vi "GUI_CameraTriggers.vi"() -> ()   [LabVIEW 2020]
uses:
  Shared/GUI_Template/GUI_master/tcp_new_data_event.ctl
  Shared/GUI_Template/GUI_master/tcp new data cluster.ctl
  <userlib>/_OpenG.lib/array/array.llb/Search 1D Array (String)__ogtk.vi
  <userlib>/_OpenG.lib/array/array.llb/Index 1D Array Elements (String)__ogtk.vi
panel:
  in  "trigger::8":bool=TRUE caption="CAM-PL1-APLSideView"
  in  "exposure::8":dbl caption="CAM-PL1-APLSideView" min=3.8e-05 max=1.0
  in  "GUIdevice 8":string="CAM-PL1-APLSideView"
  in  "trigger::2":bool=TRUE caption="1BL-M1"
  in  "exposure::2":dbl caption="1BL-M1" min=3.8e-05 max=1.0
  in  "GUIdevice 2":string="CAM-1BL-M1"
  in  "exposure::33":dbl caption="CAM-PL1-TopView" min=1.0 max=50.0
  in  "exposure::31":dbl caption="SPEC-TEA-Qred"
  in  "exposure::30":dbl caption="SPEC-AA-Hamamastsu" min=1.0 max=300.0
  in  "exposure::21":dbl caption="CAM-TEA-MagSpecL" min=0.0001 max=1.0
  in  "exposure::20":dbl caption="CAM-TEA-MagSpecK" min=0.0001 max=1.0
  in  "exposure::19":dbl caption="CAM-TEA-MagSpecD" min=0.0001 max=1.0
  in  "exposure::18":dbl caption="CAM-TEA-MagSpecJ" min=0.0001 max=1.0
  in  "exposure::16":dbl caption="CAM-TEA-MagSpecI" min=0.0001 max=1.0
  in  "exposure::15":dbl caption="CAM-TEA-MagSpecH" min=0.0001 max=1.0
  in  "exposure::14":dbl caption="CAM-TEA-MagSpecG" min=0.0001 max=1.0
  in  "exposure::13":dbl caption="CAM-TEA-MagSpecC" min=0.0001 max=1.0
  in  "exposure::12":dbl caption="CAM-TEA-MagSpecB" min=0.0001 max=1.0
  in  "exposure::11":dbl caption="CAM-TEA-MagSpecA" min=0.0001 max=1.0
  in  "exposure::10":dbl caption="CAM-TEA-EBeam_Profile" min=3e-05 max=98990.0
  in  "exposure::9":dbl caption="CAM-PL1-SideSpec" min=2.5e-05 max=1.0
  in  "exposure::7":dbl caption="CAM-PL1-APLSideView" min=3.8e-05 max=1.0
  in  "exposure::6":dbl caption="CAM-HPD-HolyWedge" min=137.0 max=1000000.0
  in  "exposure::5":dbl caption="CAM-HPD-HeatCCD" min=3.8e-05 max=1.0
  in  "exposure::4":dbl caption="CAM-HPD-CCD" min=3.8e-05 max=1.0
  in  "exposure::3":dbl caption="CAM-1BL-M5" min=3.8e-05 max=1.0
  in  "exposure::1":dbl caption="1BL-M1" min=0.001 max=1.0
  in  "Trigger.mode::29":u16(ring)=2 caption="Trigger mode" items=["Auto", "Normal", "Single", "Single, auto trigger"]
  in  "Trigger.Slope::29":u16(ring) caption="Trigger Slope" items=["Rising", "Falling"]
  in  "Trigger.Source::29":u16(ring)=1 caption="Trigger Source" items=["Channel 1", "Channel 2", "Channel 3", "Channel 4", "External", "Power Line"]
  in  "Trigger.Level::29":dbl=0.04 caption="Trigger Level (V)" min=0.0001 max=30.0 format="%#_6p"
  in  "trigger::33":bool=TRUE caption="CAM-PL1-TopView"
  in  "GUIdevice 33":string="CAM-PL1-TopView"
  in  "Trigger.Mode::26":u16(ring) caption="DAQ-AA-3" items=["Immediate", "Analog Edge", "Analog Window", "Analog Hysteresis", "Video", "Digital Edge"]
  in  "Trigger.Mode::24":u16(ring) caption="DAQ-AA-2" items=["Immediate", "Analog Edge", "Analog Window", "Analog Hysteresis", "Video", "Digital Edge"]
  in  "Trigger.Mode::22":u16(ring) caption="DAQ-AA-1" items=["Immediate", "Analog Edge", "Analog Window", "Analog Hysteresis", "Video", "Digital Edge"]
  in  "trigger::31":bool=TRUE caption="SPEC-TEA-Qred"
  in  "trigger::30":bool=TRUE caption="SPEC-AA-Hamamastsu"
  in  "trigger::21":bool=TRUE caption="CAM-TEA-MagSpecL"
  in  "trigger::20":bool=TRUE caption="CAM-TEA-MagSpecK"
  in  "trigger::19":bool=TRUE caption="CAM-TEA-MagSpecJ"
  in  "trigger::18":bool=TRUE caption="CAM-TEA-MagSpecI"
  in  "trigger::16":bool=TRUE caption="CAM-TEA-MagSpecH"
  in  "trigger::15":bool=TRUE caption="CAM-TEA-MagSpecG"
  in  "trigger::14":bool=TRUE caption="CAM-TEA-MagSpecD"
  in  "trigger::13":bool=TRUE caption="CAM-TEA-MagSpecC"
  in  "trigger::12":bool=TRUE caption="CAM-TEA-MagSpecB"
  in  "trigger::11":bool=TRUE caption="CAM-TEA-MagSpecA"
  in  "trigger::10":bool=TRUE caption="CAM-TEA-EBeam_Profile"
  in  "trigger::9":bool=TRUE caption="CAM-PL1-SideSpec"
  in  "trigger::7":bool=TRUE caption="CAM-PL1-APLSideView"
  in  "trigger::6":bool=TRUE caption="CAM-HPD-HolyWedge"
  in  "trigger::5":bool=TRUE caption="CAM-HPD-HeatCCD"
  in  "trigger::4":bool=TRUE caption="CAM-HPD-CCD"
  in  "trigger::3":bool=TRUE caption="CAM-1BL-M5"
  in  "trigger::1":bool=TRUE caption="1BL-M1"
  in  "GUIdevice 31":string="SPEC-TEA-Qred"
  in  "GUIdevice 30":string="SPEC-AA-Hamamastsu"
  in  "Jet trigger":bool caption="Triggers"
  in  "GUIdevice 4":string="CAM-HPD-CCD"
  in  "GUIdevice 6":string="CAM-HPD-HolyWedge"
  in  "GUIdevice 29":string="SCOPE-AA-LeCroy8254M"
  in  "GUIdevice 26":string="DAQ-AA-3"
  in  "GUIdevice 24":string="DAQ-AA-2"
  in  "GUIdevice 22":string="DAQ-AA-1"
  in  "GUIdevice 21":string="CAM-TEA-MagSpecL"
  in  "GUIdevice 20":string="CAM-TEA-MagSpecK"
  in  "GUIdevice 19":string="CAM-TEA-MagSpecJ"
  in  "GUIdevice 18":string="CAM-TEA-MagSpecI"
  in  "GUIdevice 16":string="CAM-TEA-MagSpecH"
  in  "GUIdevice 15":string="CAM-TEA-MagSpecG"
  out "error IO 2":errorcluster
  out "tcp data event":T1
  in  "GUIdevice 14":string="CAM-TEA-MagSpecD"
  in  "GUIdevice 13":string="CAM-TEA-MagSpecC"
  in  "GUIdevice 7":string="CAM-PL1-APLSideView"
  in  "GUIdevice 10":string="CAM-TEA-EBeam_Profile"
  in  "GUIdevice 5":string="CAM-HPD-HeatCCD"
  in  "GUIdevice 1":string="CAM-1BL-M1"
  in  "GUIdevice 3":string="CAM-1BL-M5"
  in  "GUIdevice 11":string="CAM-TEA-MagSpecA"
  in  "GUIdevice 12":string="CAM-TEA-MagSpecB"
  in  "GUIdevice 9":string="CAM-PL1-SideSpec"
  in  "stop":bool
  # "CAM-1BL-CompG4\n\nCAM-1BL-M1back\n\n\n\nCAM-2BL-GHOST\n\n\n\nCAM-HPD-CCD2\nCAM-HPD-CCD3\n\nCAM-HPD-HeatM3\n\n\nCAM-LT-SPLIT\nCAM-LT-XPW\n\nCAM-PL1-LPMode\nCAM-PL1-PMReflect\n\nCAM-PL1-SideSpec\nCAM-PL1-SideView\nCAM-PL1-TopView\n\n\n\n\n\n\n\n\nCAM-TEA-MagSpecHR\n\n\n\n\n\n\n\nEM-HPD-1\nEM-LB-1\nEM-LB-1\nEM-LB-PL\nFROG-HPD-1\nFROG-LB-1\nHPD-Phasics151\nIP2-MCPcam\nIP2-modeim\nIP2-Reflected1\nIP2-Reflected1\nIP2-targetobs\nIP2-targetscatt\nIP2-transmit\nP2-AndorCam\nP2-DG535\nP2-HeatCamPost\nP2-HeatCamPostNear\nP2-HeatCamPreFar\nP2-HeatCamPreNear\nP2-HeatCamPreNear\nP2-HeatEnergy\nP2-HeatEnergy\nP2-phasics\nP2-phasicsHR\nP2-ProbeCamPost\nP2-ProbeCamPostNear\nP2-ProbeCamPreNear\nP2-SideView\nP2-SRS\nP2-SRS\nP2FastDiag645\nP2FastDiag645\n\nSCOPE-LT-LeCroy64Xi\nSCOPE-PL1-PXIfast\nSCOPE-PL1-PXIfast\nSCOPE-PL1-PXIfast\nSCOPE-PL1-PXIfast\nSPEC-AA-Hamamastsu\nSPEC-PL1-Thorlabs\nSPEC-TEA-Qred"
  # "BELLA Triggers"
  # "SCOPE-AA-LeCroy8254M"
  # "Trigger"
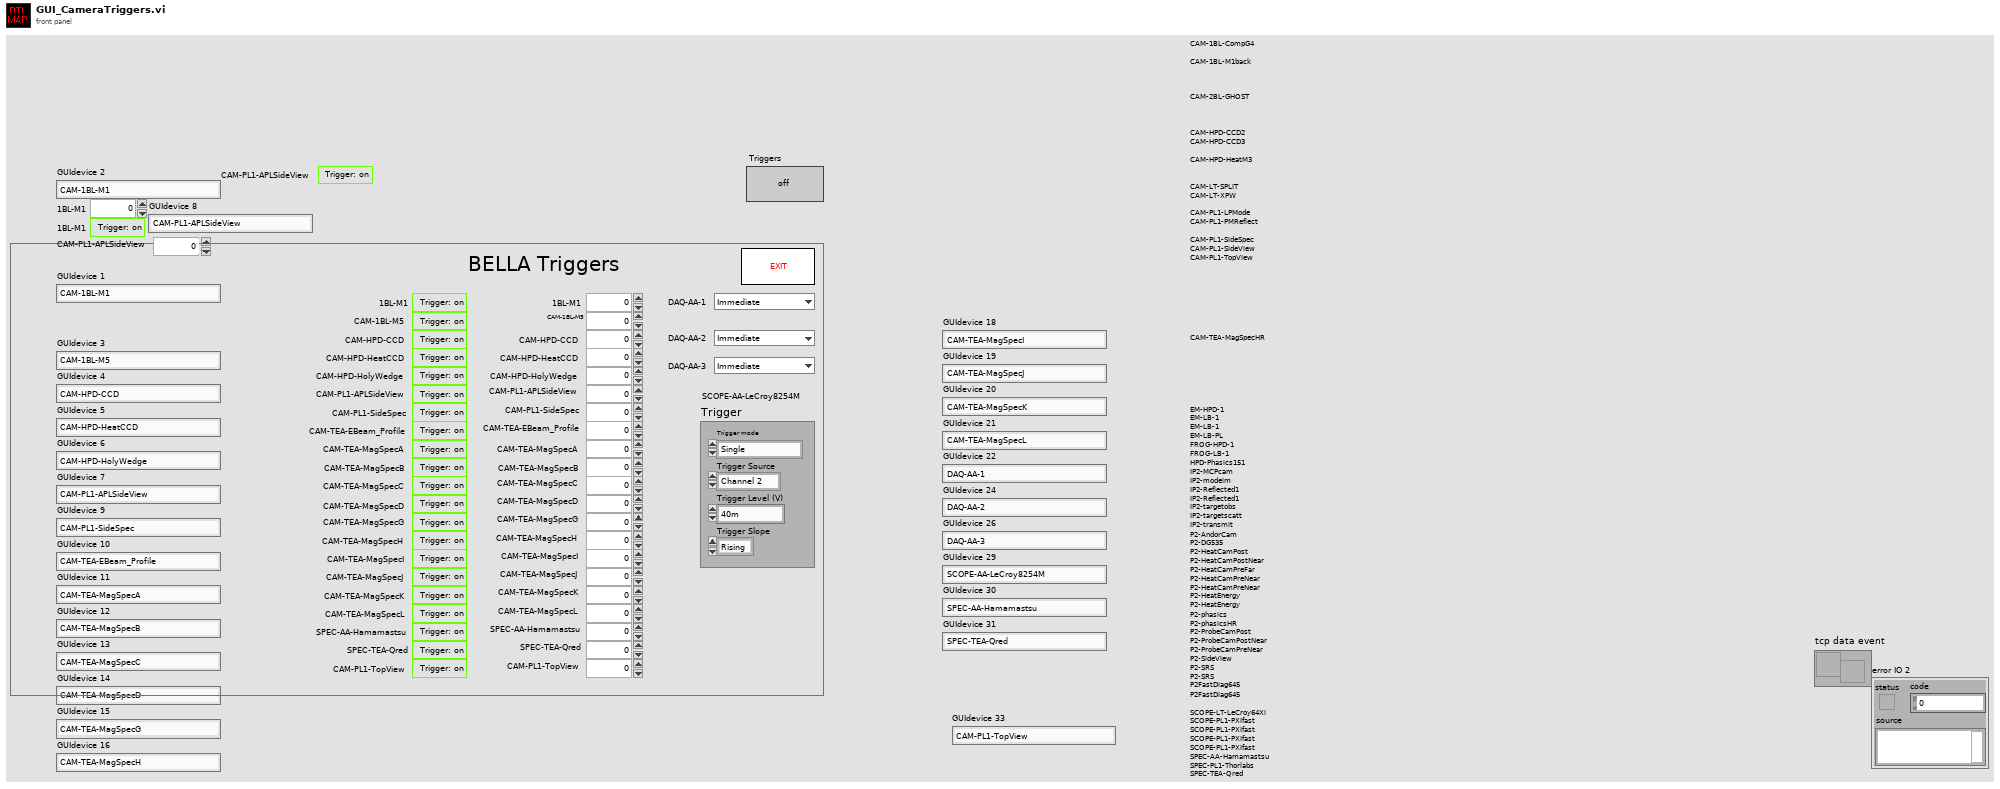
[diagram p1: front panel]
types:
  T1 = typedef "tcp_new_data_event.ctl" = refnum<user-event>
  T2 = typedef "tcp new data cluster.ctl" = cluster{"EventEnum":enum16{"new data", "connection status update"}, "Device name":string}
  T3 = enum32{"invalid app kind", "Development System", "Run Time System", "Student Edition", "Embedded LabVIEW", "Evaluation", "Custom"}
  T4 = enum32{"Invalid", "Standard", "Closed", "Hidden", "Minimized", "Maximized"}
  T5 = cluster{"Core":cluster{"Current VI Reference":refnum<vi>, "Close Panel on Exit?":bool}, "Heater timing offset":dbl, "Discharge timing offset":dbl, "Jet trigger":bool, "Tik1":u32, "Tik2":u32, "Fire Continues Allowed":bool}
  T6 = cluster{"Current VI Reference":refnum<vi>, "Close Panel on Exit?":bool}
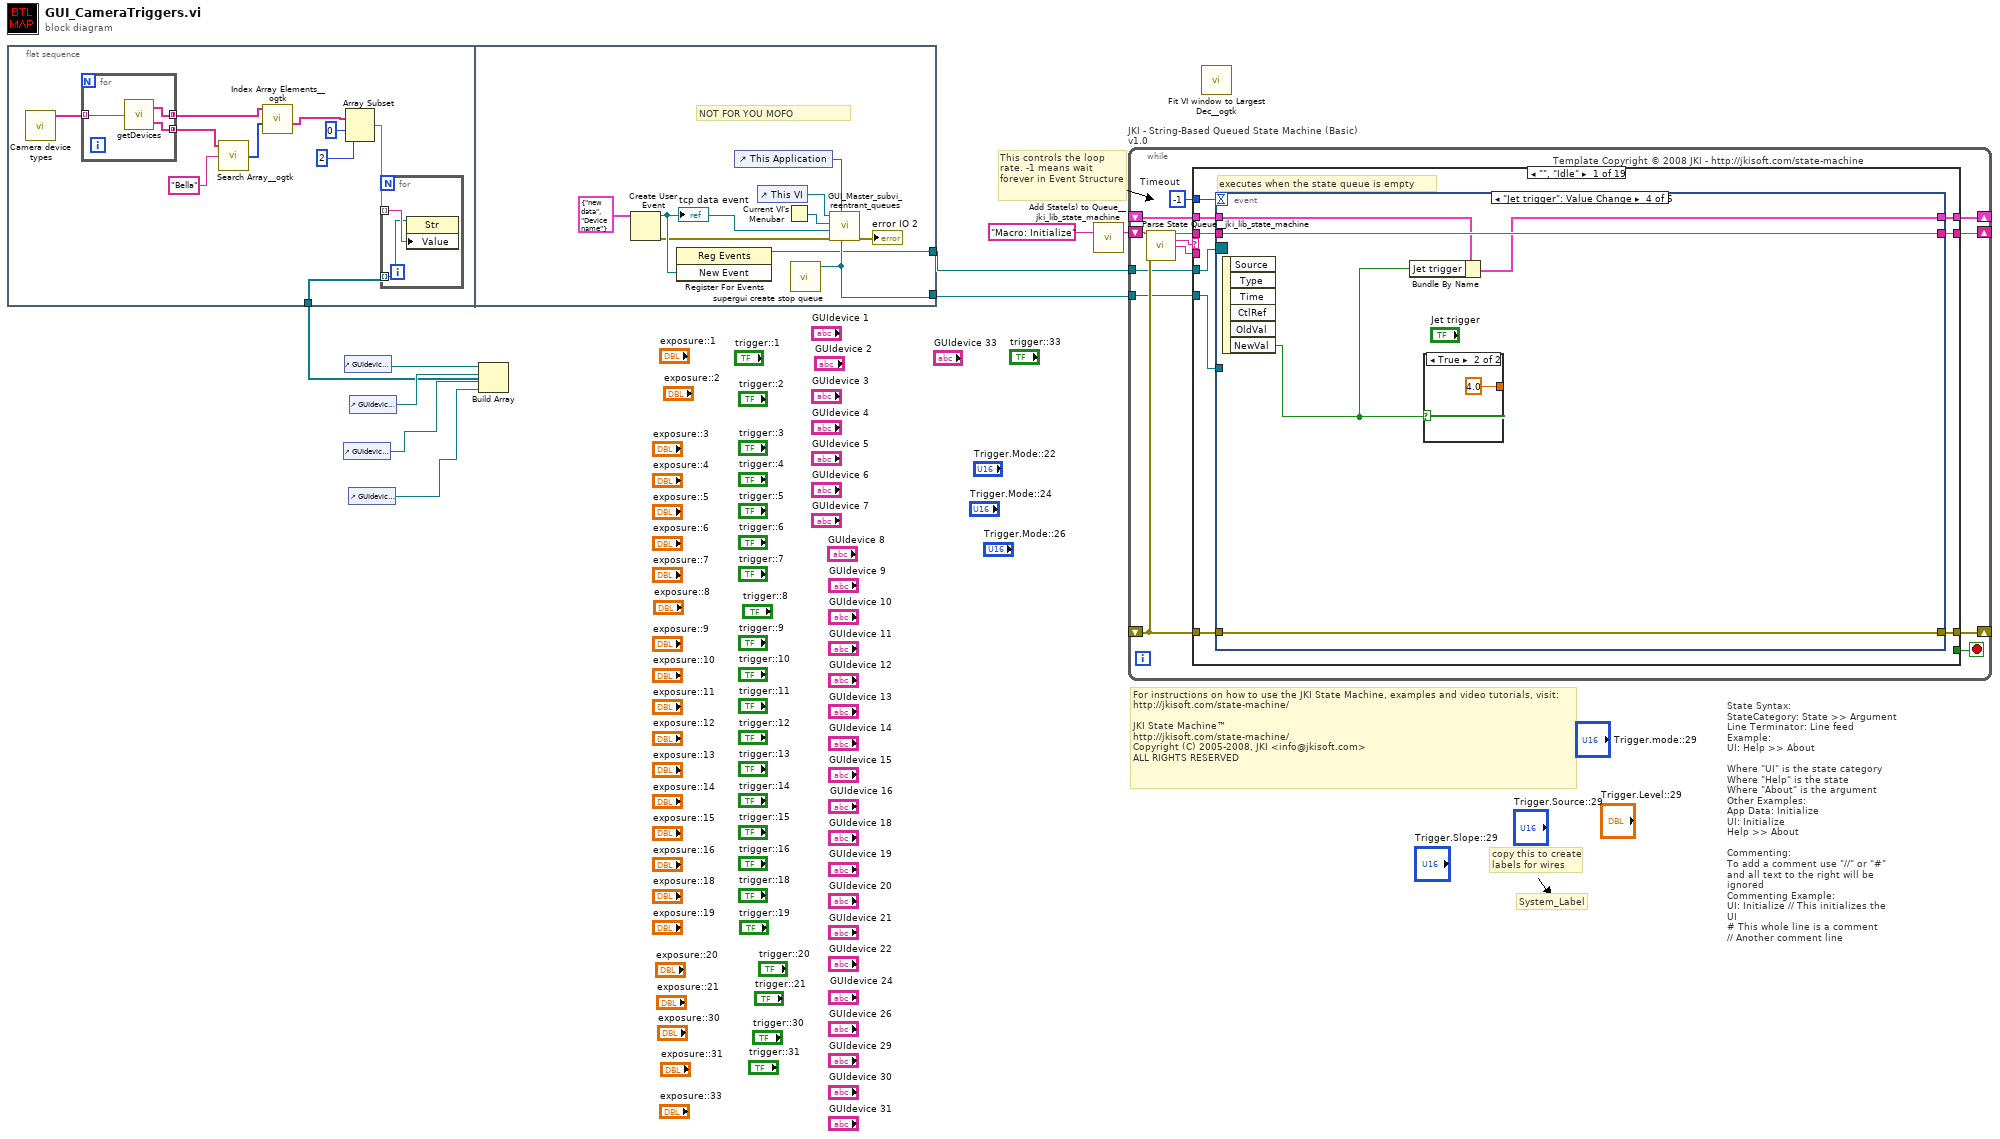
[diagram p0: block diagram]
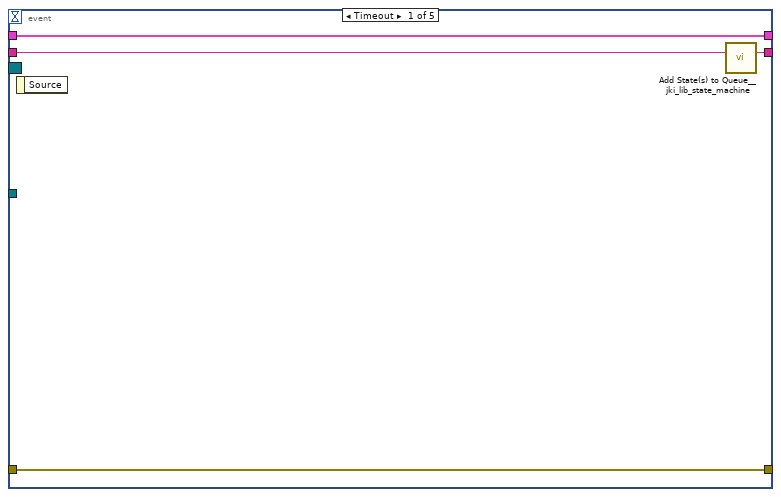
[diagram p2: hidden frame]
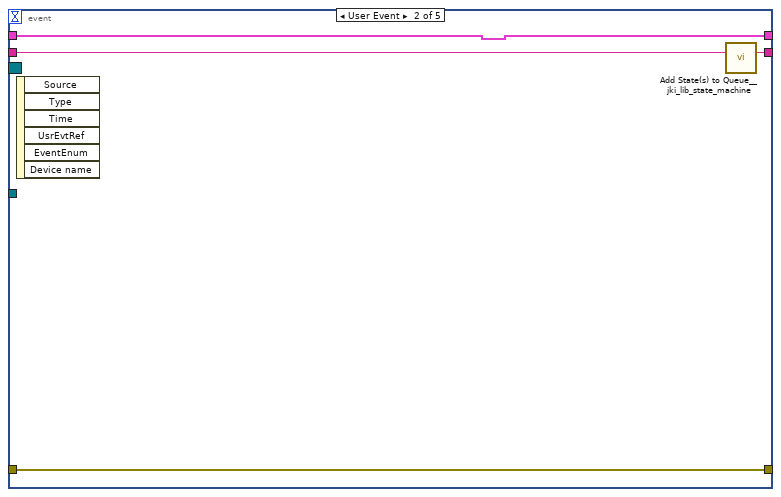
[diagram p3: hidden frame]
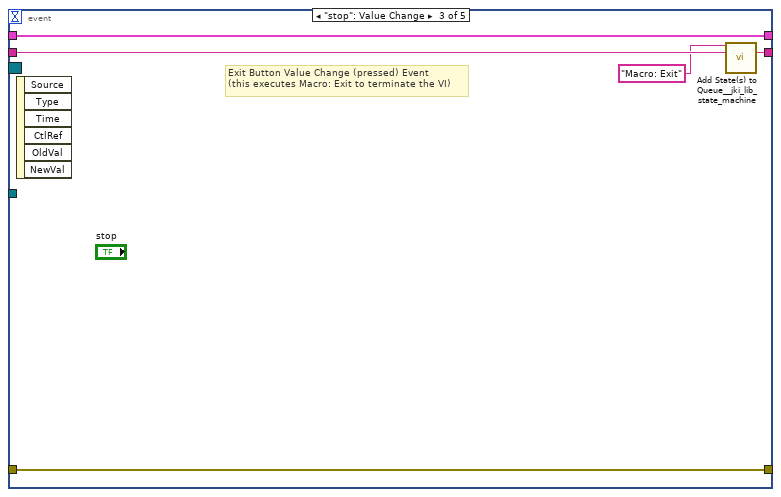
[diagram p4: hidden frame]
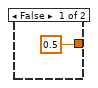
[diagram p5: hidden frame]
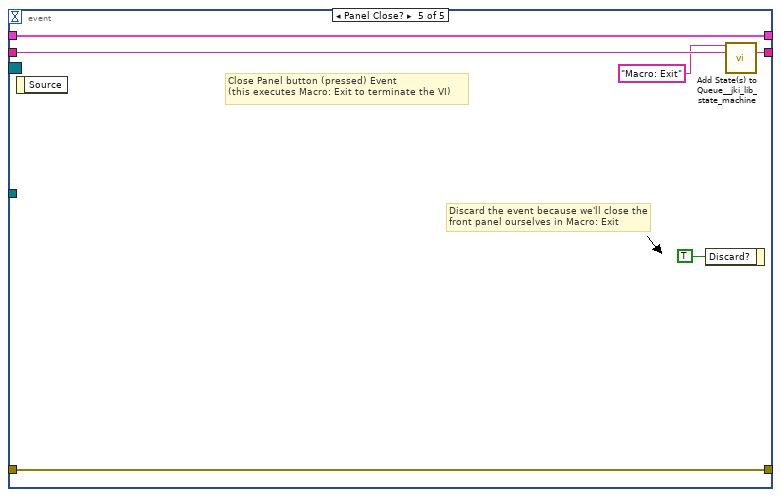
[diagram p6: hidden frame]
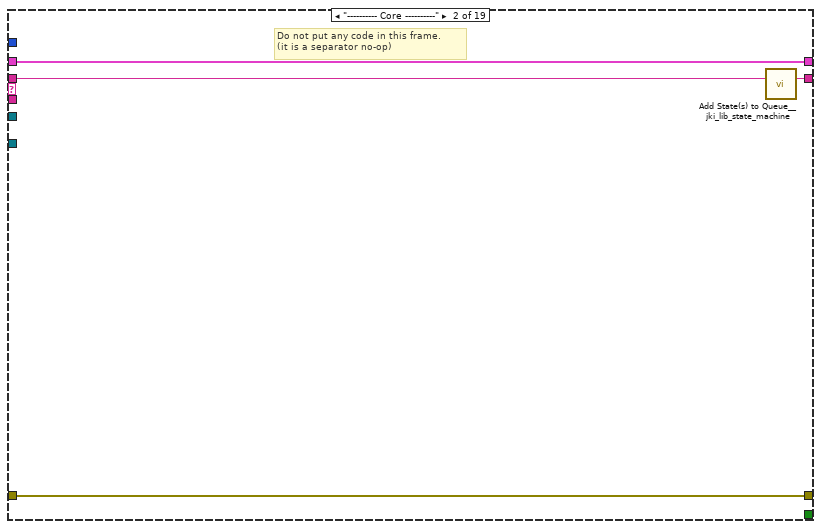
[diagram p7: hidden frame]
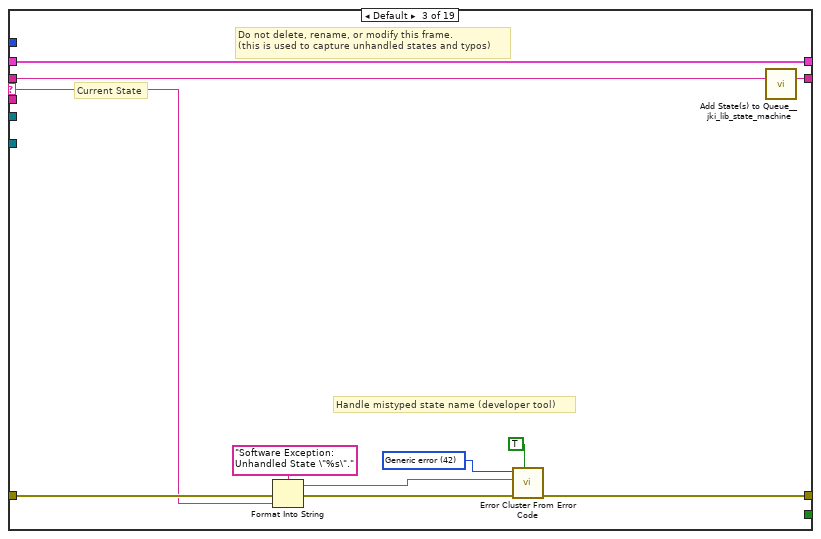
[diagram p8: hidden frame]
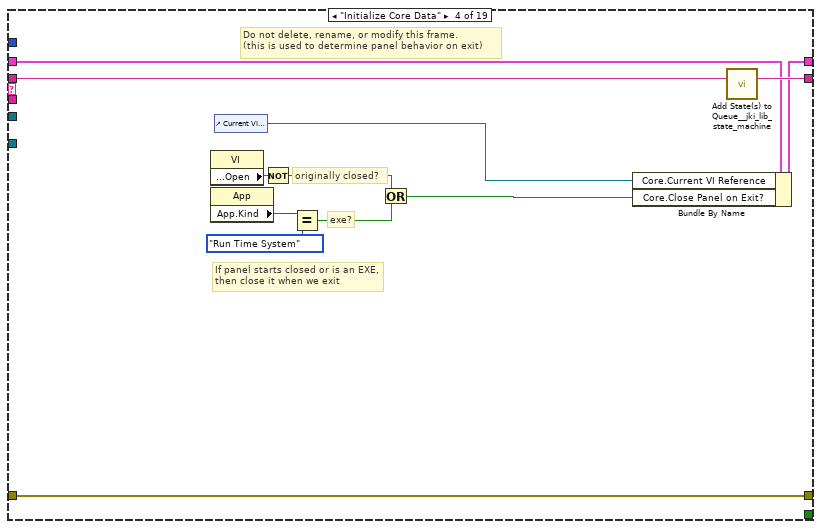
[diagram p9: hidden frame]
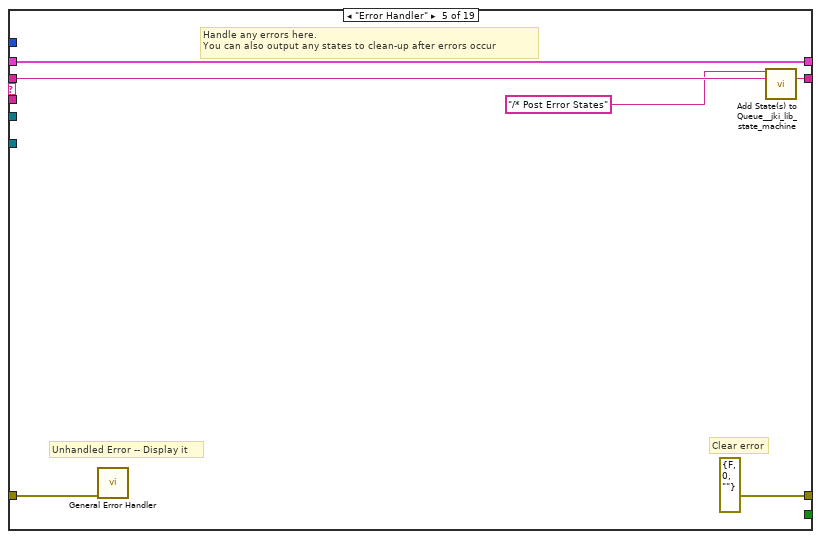
[diagram p10: hidden frame]
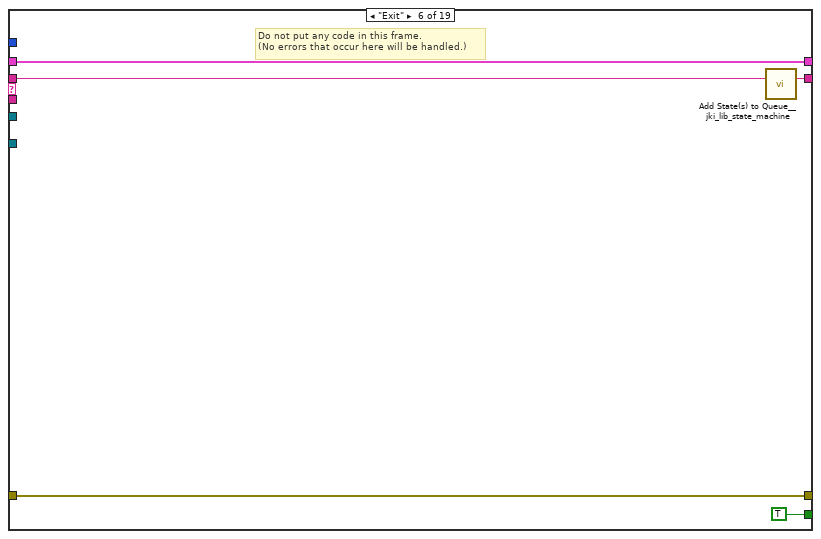
[diagram p11: hidden frame]
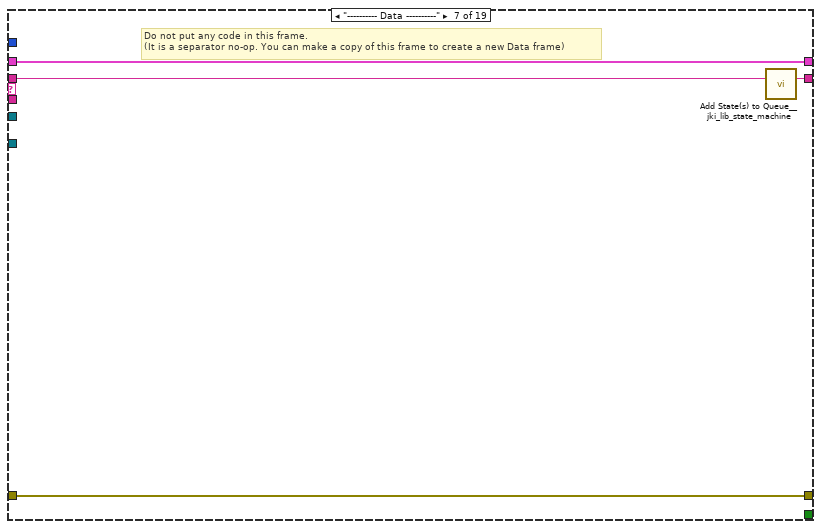
[diagram p12: hidden frame]
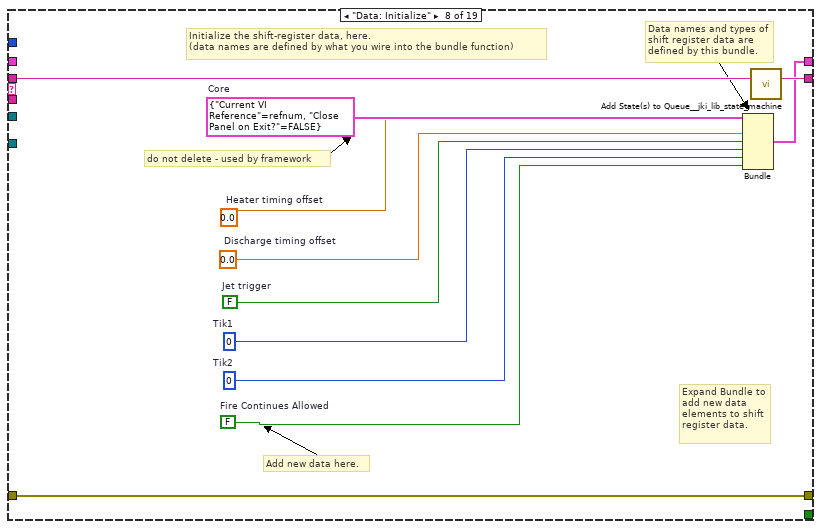
[diagram p13: hidden frame]
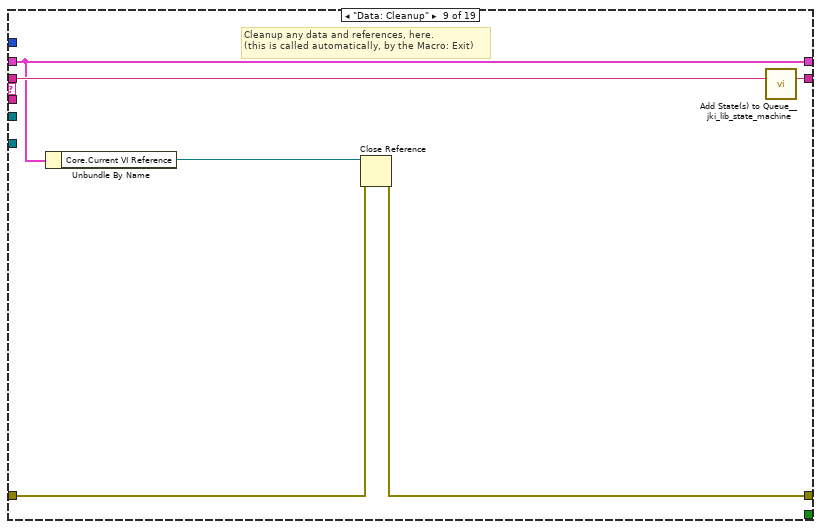
[diagram p14: hidden frame]
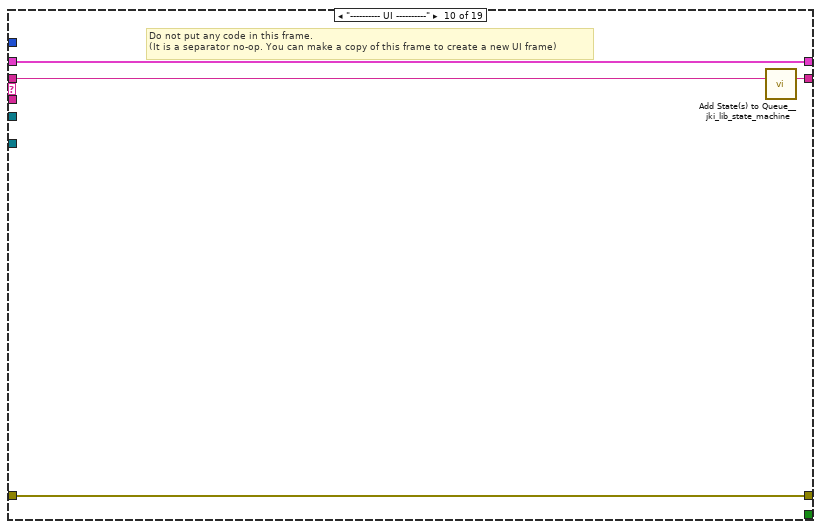
[diagram p15: hidden frame]
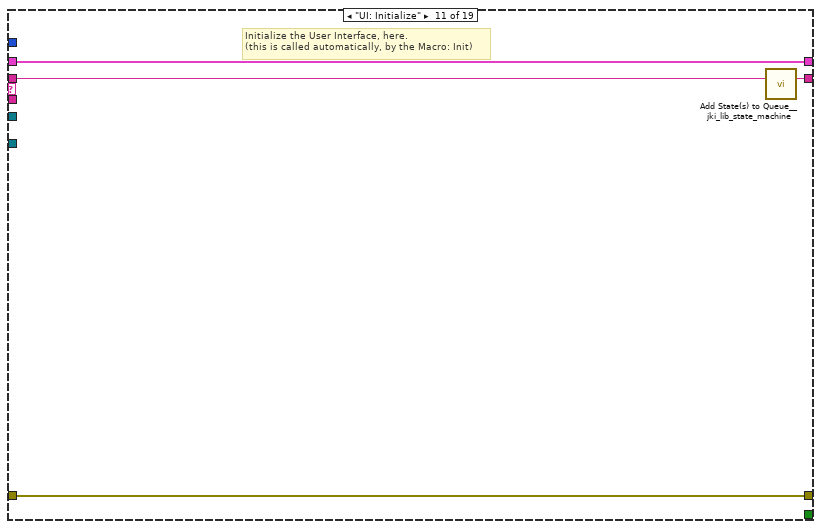
[diagram p16: hidden frame]
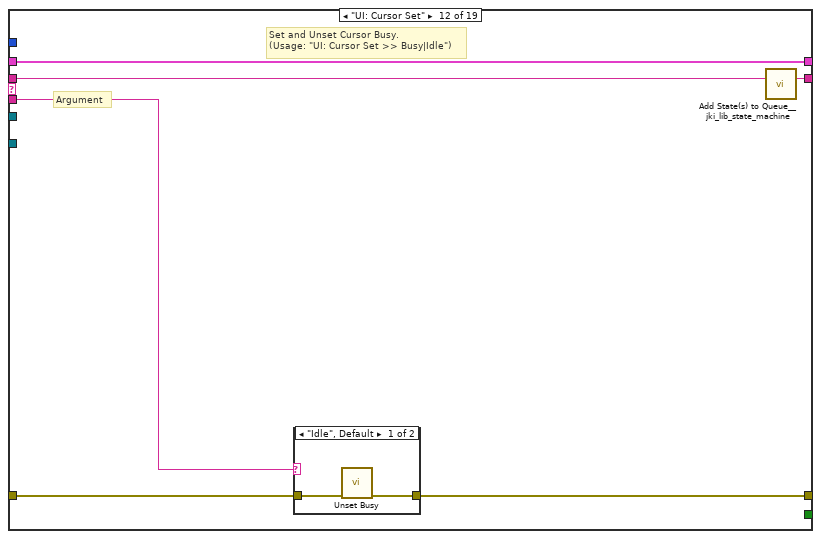
[diagram p17: hidden frame]
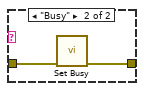
[diagram p18: hidden frame]
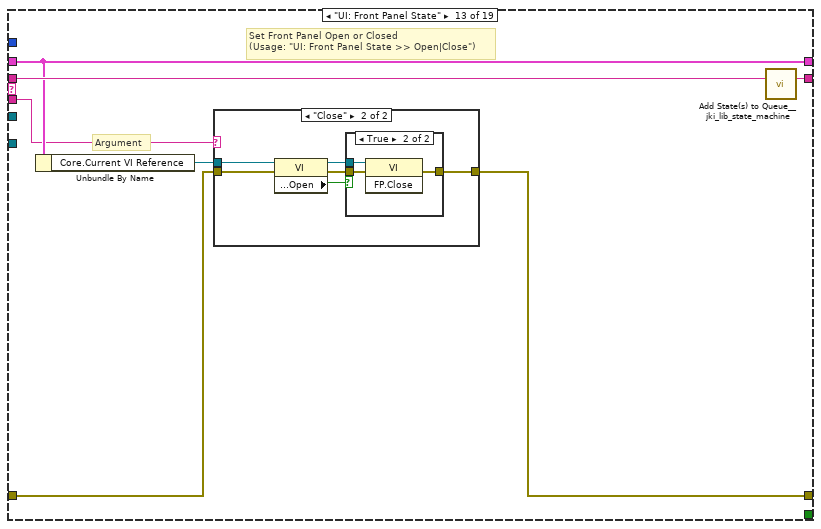
[diagram p19: hidden frame]
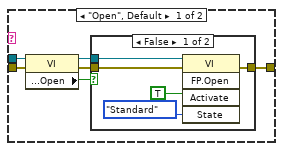
[diagram p20: hidden frame]
diagram:
  # "For instructions on how to use the JKI State Machine, examples and video tutorials, visit:\nhttp://jkisoft.com/state-machine/\n\nJKI State Machine™\nhttp://jkisoft.com/state-machine/\nCopyright (C) 2005-2008, JKI <info@jkisoft.com>\nALL RIGHTS RESERVED"
  # "State Syntax:\nStateCategory: State >> Argument\nLine Terminator: Line feed\nExample:\nUI: Help >> About\n\nWhere \"UI\" is the state category\nWhere \"Help\" is the state\nWhere \"About\" is the argument\nOther Examples:\nApp Data: Initialize\nUI: Initialize\nHelp >> About\n\nCommenting:\nTo add a comment use \"//\" or \"#\" and all text to the right will be ignored\nCommenting Example:\nUI: Initialize // This initializes the UI\n# This whole line is a comment\n// Another comment line"
  # "copy this to create labels for wires"
  # "This controls the loop rate. -1 means wait forever in Event Structure"
  # "System_Label"
  n1 = flat-sequence {
    tunnel: w1 -> [w15]
    tunnel: [w26] -> w7
    tunnel: [w25] -> w6
    frame #0 {
      n2 = call "Camera device types.vi"() -> ("Camera device types"=w19:string[])  [unwired: 11 in]
      n3 = for {
        tunnel: [w24] -> w12 mode=concatenating
        tunnel: w19 -> [w23] mode=indexing
        tunnel: [w22] -> w14 mode=concatenating
        n4 = call "getDevices.vi"("Device Class"=w23) -> ("All Devices"=w24:string[], "Expts"=w22:string[])
      }
      n5 = call-poly <userlib>:"Search Array__ogtk.vi"("Array"=w14, "Element Data"="Bella") -> ("Indices of Elements"=w11:i32[])  [unwired: 7 in]
      n6 = call-poly <userlib>:"Index Array Elements__ogtk.vi"("indices"=w11, "array"=w12) -> ("elements"=w10:string[])  [unwired: 9 in]
      n7 = Array Subset(array=w10, index=0, length=2) -> (w16:string[])
      n8 = for {
        tunnel: w16 -> [w21] mode=indexing
        tunnel: w15 -> [w20] mode=indexing
        n9 = property on="Property Node" class="Str"(reference=w20, "Value"=w21) -> ()  [unwired: 1 in, 2 out]
      }
    }
    frame #1 {
      # "NOT FOR YOU MOFO"
      n10 = Create User Event(user event datatype=T2 {"EventEnum"=enum."new data", "Device name"="Device name"} ("New Event")) -> (user event=w32:refnum<user-event>, error out=w31:errorcluster)  [unwired: 1 in]
      "tcp data event" <- w32
      n11 = register-events(w32) -> (reference out=w25:refnum<event-registration>)  [unwired: 2 in, 1 out]
      n12 = control-ref of="This Application"() -> (w33:refnum<vi>)
      n13 = control-ref of="This VI"() -> (w27:refnum<vi>)
      n14 = Current VI's Menubar() -> (w29:refnum<k9>)
      n15 = call "supergui create stop queue.vi"() -> ("STOP Queue out"=w26:refnum<queue>)  [unwired: 11 in]
      n16 = call "GUI_Master_subvi_reentrant_queues.vi"("STOP Queue in"=w26, "This Application"=w33, "error in (no error)"=w31, "tcp data event"=w32, "Caller menu reference"=w29, "Caller VI ref"=w27) -> ("error out"=→"error IO 2":errorcluster)  [unwired: 5 in]
    }
  }
  n17 = control-ref of="GUIdevice 3"() -> (w3:refnum<vi>)
  n18 = control-ref of="GUIdevice 1"() -> (w5:refnum<vi>)
  n19 = control-ref of="GUIdevice 4"() -> (w2:refnum<vi>)
  n20 = control-ref of="GUIdevice 2"() -> (w4:refnum<vi>)
  n21 = Build Array(w5, w4, w3, w2) -> (w1:refnum<vi>[])
  n22 = call <vilib>:"Add State(s) to Queue__jki_lib_state_machine.vi"("State(s) in (\"\")"="Macro: Initialize") -> ("States Out"=w8:string)  [unwired: 14 in]
  n23 = while "JKI - String-Based Queued State Machine (Basic) v1.0" {
    shift-right: [w39] -> _
    shift-left: _ -> [w38]
    shift-right: [w42] -> _
    shift-left: _ -> [w36]
    shift-right: [w41] -> _
    shift-left: w8 -> [w43]
    tunnel: w6 -> [w35]
    tunnel: w7 -> [w34]
    stop <- w40 stop-if-true
    w37 = -1  # Timeout
    # "Template Copyright © 2008 JKI - http://jkisoft.com/state-machine"
    n24 = call <vilib>:"Parse State Queue__jki_lib_state_machine.vi"("State Queue"=w43, "Error In (no error)"=w36) -> ("Remaining States"=w45:string, "Current State"=w46:string, "Arguments"=w44:string)  [unwired: 11 in]
    n25 = case shown="\"\", \"Idle\"" w46 {
      selector: w46 -> [_ _ w86 _ _ _ _ _ _ _ _ _ _ _ _ _ _ _ _]
      tunnel: w45 -> [w55 w85 w90 w108 w114 w119 w123 w134 w140 w144 w148 w154 w165 w191 w196 w209 w213 w225 w232]
      tunnel: w44 -> [_ _ _ _ _ _ _ _ _ _ _ w149 w159 _ _ _ _ _ _]
      tunnel: w38 -> [w53 w82 w88 w99 w111 w117 w120 _ w135 w141 w146 w152 w161 w188 w193 w206 w210 w222 w230]
      tunnel: [w52 w83 w92 w105 errorcluster {"status"=FALSE, "code"=0, "source"=""} ("error out") w116 w121 w131 w136 w142 w145 w150 w162 w189 w194 w207 w211 w223 w229] -> w42
      tunnel: w36 -> [w51 w83 w91 w105 w110 w116 w121 w131 w137 w142 w145 w151 w163 w189 w194 w207 w211 w223 w229]
      tunnel: [w54 w84 w89 w107 w113 w118 w122 w133 w139 w143 w147 w153 w164 w190 w195 w208 w212 w224 w231] -> w41
      tunnel: [_ _ _ _ _ TRUE _ _ _ _ _ _ _ _ _ _ _ _ _] -> w40
      tunnel: [w47 w82 w88 w106 w111 w117 w120 w132 w135 w141 w146 w152 w161 w188 w193 w206 w210 w221 w230] -> w39
      tunnel: w37 -> [w50 _ _ _ _ _ _ _ _ _ _ _ _ _ _ _ _ _ _]
      tunnel: w35 -> [w49 _ _ _ _ _ _ _ _ _ _ _ _ _ _ _ _ _ _]
      tunnel: w34 -> [w48 _ _ _ _ _ _ _ _ _ _ _ _ _ _ w198 _ _ _]
      frame "", "Idle" {
        # "executes when the state queue is empty"
        n26 = event shown="[3] \"Jet trigger\": Value Change" {
          selector: w49 -> [_ _ _ _ _]
          dyn-events: _ -> [_ _ _ _ _]
          timeout: w50 -> [_ _ _ _ _]
          tunnel: w55 -> [w59 w63 w68 w73 w81]
          tunnel: [w58 w62 w67 w73 w80] -> w54
          tunnel: w53 -> [w56 w60 w65 w72 w78]
          tunnel: [w57 w61 w66 w69 w79] -> w52
          tunnel: w51 -> [w57 w61 w66 w69 w79]
          tunnel: [w56 w60 w65 w71 w78] -> w47
          tunnel: w48 -> [_ _ _ _ _]
          event Timeout {
            n27 = event-data() -> ()  [unwired: 1 in, 1 out]
            n28 = call <vilib>:"Add State(s) to Queue__jki_lib_state_machine.vi"("State(s) in (\"\")"=w59) -> ("States Out"=w58:string)  [unwired: 14 in]
          }
          event User Event {
            n29 = event-data() -> ()  [unwired: 1 in, 6 out]
            n30 = call <vilib>:"Add State(s) to Queue__jki_lib_state_machine.vi"("State(s) in (\"\")"=w63) -> ("States Out"=w62:string)  [unwired: 14 in]
          }
          event "stop": Value Change {
            # "Exit Button Value Change (pressed) Event\n(this executes Macro: Exit to terminate the VI)"
            n31 = event-data() -> ()  [unwired: 1 in, 6 out]
            n32 = call <vilib>:"Add State(s) to Queue__jki_lib_state_machine.vi"("State(s) in Front (\"\")"="Macro: Exit", "State(s) in (\"\")"=w68) -> ("States Out"=w67:string)  [unwired: 13 in]
          }
          event "Jet trigger": Value Change {
            n33 = event-data() -> ("NewVal"=w70:bool)  [unwired: 1 in, 5 out]
            n34 = Bundle By Name(cluster=w72, "Jet trigger"=w70) -> (w71:T5)
            n35 = case shown="True" w70 {
              tunnel: [0.5 ("Amplitude.Ch CD::10") 4.0 ("Amplitude.Ch CD::10")] -> _
              frame False {
              }
              frame True {
              }
            }
          }
          event Panel Close? {
            # "Discard the event because we'll close the front panel ourselves in Macro: Exit"
            # "Close Panel button (pressed) Event\n(this executes Macro: Exit to terminate the VI)"
            n36 = event-data() -> ()  [unwired: 1 in, 1 out]
            n37 = event-data("Discard?"=TRUE) -> ()  [unwired: 1 in, 1 out]
            n38 = call <vilib>:"Add State(s) to Queue__jki_lib_state_machine.vi"("State(s) in Front (\"\")"="Macro: Exit", "State(s) in (\"\")"=w81) -> ("States Out"=w80:string)  [unwired: 13 in]
          }
        }
      }
      frame "---------- Core ----------" {
        # "Do not put any code in this frame.\n(it is a separator no-op)"
        n39 = call <vilib>:"Add State(s) to Queue__jki_lib_state_machine.vi"("State(s) in (\"\")"=w85) -> ("States Out"=w84:string)  [unwired: 14 in]
      }
      frame Default {
        w95 = 42 items=["No error", "Argument error", "Memory is full", "Out of zone", "End of file", "File already open", "Generic file I/O error", "File not found", "File permission error", "Disk is full", "Duplicate path", "Too many files open", "System feature not enabled", "Resource file not found", "Cannot add resource", "Resource not found", "Image not found", "Image memory error", "Pen does not exist", "Config type invalid", "Config token not found", "Config parse error", "Config memory error", "Bad external code format", "Bad external code offset", "External code not present", "Null window", "Destroy window error", "Null menu", "Print aborted", "Bad print record", "Print driver error", "Windows error during printing", "Memory error during printing", "Print dialog error", "Generic print error", "Invalid device refnum", "Device not found", "Device parameter error", "Device unit error", "Cannot open device", "Device call aborted", "Generic error", "Cancelled by user", "Object ID too low", "Object ID too high", "Object not in heap", "Unknown heap", "Unknown object (invalid DefProc)", "Unknown object (DefProc not in table)", "Message out of range", "Invalid (null) method", "Unknown message", "Manager call not supported", "Bad address", "Network operation in progress", "Network operation timed out", "Connection is busy", "Network attribute not supported", "Network error", "Address in use", "System out of memory", "Connection aborted", "Connection refused", "Not connected", "Already connected", "Connection closed", "Initialization error (interapplication manager)", "Bad occurrence", "Wait on unbound occurrence handler", "Occurrence queue overflow", "Datalog type conflict", "Unused", "Unrecognized type (interapplication manager)", "Memory corrupt", "Failed to make temporary DLL", "Old CIN version", "Drag socket not found", "Failed to load drop-object", "Failed to register OLE object", "Failed to release OLE object", "Format specifier type mismatch", "Unknown format specifier", "Too few format specifiers", "Too many format specifiers", "Scan failed", "Newer CIN version", "Error converting to variant", "Runtime menu error", "Password tampered", "Variant attribute not found", "Incompatible variant data type", "Event data is not available", "Event Store is not present", "Occurrence is not found", "Event Queue is not created", "Event info is not available", "Refnum passed is NULL", "Error retrieving Class GUID", "Error retrieving CoClass GUID", "Error retrieving TypeLib GUID.", "Bad built application magic bytes.", "Specific driver is different from the specific driver associated with the Logical Name.", "There is no session opened to the class driver.", "Max Error", "MAX - Error with config objects", "MAX - Error loading configuration", "MAX - Group not supported"]
        # "Current State"
        # "Do not delete, rename, or modify this frame.\n(this is used to capture unhandled states and typos)"
        # "Handle mistyped state name (developer tool)"
        n40 = Format Into String(format string="Software Exception: Unhandled State \"%s\"." ("message"), error in=w91, w86) -> (resulting string=w94:string, error out=w93:errorcluster)  [unwired: 1 in]
        n41 = call <vilib>:"Error Cluster From Error Code.vi"("show call chain? (False)"=TRUE, "error in (no error)"=w93, "error message (\"\")"=w94, "error code (0)"=w95) -> ("error out"=w92:errorcluster)  [unwired: 5 in]
        n42 = call <vilib>:"Add State(s) to Queue__jki_lib_state_machine.vi"("State(s) in (\"\")"=w90) -> ("States Out"=w89:string)  [unwired: 14 in]
      }
      frame "Initialize Core Data" {
        # "Do not delete, rename, or modify this frame.\n(this is used to determine panel behavior on exit)"
        # "originally closed?"
        # "exe?"
        # "If panel starts closed or is an EXE, then close it when we exit"
        n43 = property class="VI"() -> ("Front Panel.Open"=w104:bool)  [unwired: 2 in, 2 out]
        n44 = property class="App"() -> ("App.Kind"=w103:T3)  [unwired: 2 in, 2 out]
        n45 = control-ref of="Current VI Reference"() -> (w97:refnum<vi>)
        n46 = Not(x=w104) -> (.not. x?=w101:bool)
        n47 = Equal?(x=w103, y=T3."Run Time System" ("Application:Kind")) -> (x = y?=w100:bool)
        n48 = Or(x=w101, y=w100) -> (x .or. y?=w98:bool)
        n49 = Bundle By Name(cluster=w99, "Core.Current VI Reference"=w97, "Core.Close Panel on Exit?"=w98) -> (w106:T5)
        n50 = call <vilib>:"Add State(s) to Queue__jki_lib_state_machine.vi"("State(s) in (\"\")"=w108) -> ("States Out"=w107:string)  [unwired: 14 in]
      }
      frame "Error Handler" {
        # "Unhandled Error -- Display it"
        # "Handle any errors here.\nYou can also output any states to clean-up after errors occur"
        # "Clear error"
        n51 = call <vilib>:"General Error Handler.vi"("error in (no error)"=w110) -> ()  [unwired: 10 in, 5 out]
        n52 = call <vilib>:"Add State(s) to Queue__jki_lib_state_machine.vi"("State(s) in Front (\"\")"="/* Post Error States", "State(s) in (\"\")"=w114) -> ("States Out"=w113:string)  [unwired: 13 in]
      }
      frame "Exit" {
        # "Do not put any code in this frame.\n(No errors that occur here will be handled.)"
        n53 = call <vilib>:"Add State(s) to Queue__jki_lib_state_machine.vi"("State(s) in (\"\")"=w119) -> ("States Out"=w118:string)  [unwired: 14 in]
      }
      frame "---------- Data ----------" {
        # "Do not put any code in this frame.\n(It is a separator no-op. You can make a copy of this frame to create a new Data frame)"
        n54 = call <vilib>:"Add State(s) to Queue__jki_lib_state_machine.vi"("State(s) in (\"\")"=w123) -> ("States Out"=w122:string)  [unwired: 14 in]
      }
      frame "Data: Initialize" {
        w124 = FALSE  # Fire Continues Allowed
        w126 = u32 0  # Tik1
        w125 = u32 0  # Tik2
        w127 = FALSE  # Jet trigger
        w128 = 0.0  # Discharge timing offset
        w129 = 0.0  # Heater timing offset
        w130 = T6 {"Current VI Reference"=refnum, "Close Panel on Exit?"=FALSE}  # Core
        # "do not delete - used by framework"
        # "Expand Bundle to add new data elements to shift register data."
        # "Add new data here."
        # "Data names and types of shift register data are defined by this bundle."
        # "Initialize the shift-register data, here.\n(data names are defined by what you wire into the bundle function)"
        n55 = Bundle("Core"=w130, "Heater timing offset"=w129, "Discharge timing offset"=w128, "Jet trigger"=w127, "Tik1"=w126, "Tik2"=w125, "Fire Continues Allowed"=w124) -> (w132:T5)  [unwired: 1 in]
        n56 = call <vilib>:"Add State(s) to Queue__jki_lib_state_machine.vi"("State(s) in (\"\")"=w134) -> ("States Out"=w133:string)  [unwired: 14 in]
      }
      frame "Data: Cleanup" {
        # "Cleanup any data and references, here.\n(this is called automatically, by the Macro: Exit)"
        n57 = Unbundle By Name(w135) -> ("Core.Current VI Reference"=w138:refnum<vi>)
        n58 = Close Reference(reference=w138, error in (no error)=w137) -> (error out=w136:errorcluster)
        n59 = call <vilib>:"Add State(s) to Queue__jki_lib_state_machine.vi"("State(s) in (\"\")"=w140) -> ("States Out"=w139:string)  [unwired: 14 in]
      }
      frame "---------- UI ----------" {
        # "Do not put any code in this frame.\n(It is a separator no-op. You can make a copy of this frame to create a new UI frame)"
        n60 = call <vilib>:"Add State(s) to Queue__jki_lib_state_machine.vi"("State(s) in (\"\")"=w144) -> ("States Out"=w143:string)  [unwired: 14 in]
      }
      frame "UI: Initialize" {
        # "Initialize the User Interface, here.\n(this is called automatically, by the Macro: Init)"
        n61 = call <vilib>:"Add State(s) to Queue__jki_lib_state_machine.vi"("State(s) in (\"\")"=w148) -> ("States Out"=w147:string)  [unwired: 14 in]
      }
      frame "UI: Cursor Set" {
        # "Argument"
        # "Set and Unset Cursor Busy.\n(Usage: \"UI: Cursor Set >> Busy|Idle\")"
        n62 = case shown="\"Idle\", Default" w149 {
          tunnel: w151 -> [w156 w158]
          tunnel: [w155 w157] -> w150
          frame "Idle", Default {
            n63 = call <vilib>:"Unset Busy.vi"("error in (no error)"=w156) -> ("error out"=w155:errorcluster)  [unwired: 10 in]
          }
          frame "Busy" {
            n64 = call <vilib>:"Set Busy.vi"("error in (no error)"=w158) -> ("error out"=w157:errorcluster)  [unwired: 9 in, 1 out]
          }
        }
        n65 = call <vilib>:"Add State(s) to Queue__jki_lib_state_machine.vi"("State(s) in (\"\")"=w154) -> ("States Out"=w153:string)  [unwired: 14 in]
      }
      frame "UI: Front Panel State" {
        # "Argument"
        # "Set Front Panel Open or Closed\n(Usage: \"UI: Front Panel State >> Open|Close\")"
        n66 = Unbundle By Name(w161) -> ("Core.Current VI Reference"=w160:refnum<vi>)
        n67 = case shown="\"Close\"" w159 {
          tunnel: w163 -> [w169 w182]
          tunnel: [w171 w183] -> w162
          tunnel: w160 -> [w170 w180]
          frame "Open", Default {
            n68 = property class="VI"(reference=w170, error in=w169) -> (reference out=w167:refnum<vi>, error out=w168:errorcluster, "Front Panel.Open"=w166:bool)
            n69 = case shown="False" w166 {
              tunnel: [w174 w177] -> w171
              tunnel: w168 -> [w173 w177]
              tunnel: w167 -> [w172 _]
              frame False {
                n70 = invoke class="VI" method="FP.Open"(reference=w172, error in=w173, "Activate"=TRUE, "State"=T4."Standard") -> (error out=w174:errorcluster)  [unwired: 1 in, 4 out]
              }
              frame True {
              }
            }
          }
          frame "Close" {
            n71 = property class="VI"(reference=w180, error in=w182) -> (reference out=w179:refnum<vi>, error out=w181:errorcluster, "Front Panel.Open"=w178:bool)
            n72 = case shown="True" w178 {
              tunnel: [w184 w187] -> w183
              tunnel: w181 -> [w184 w186]
              tunnel: w179 -> [_ w185]
              frame False {
              }
              frame True {
                n73 = invoke class="VI" method="FP.Close"(reference=w185, error in=w186) -> (error out=w187:errorcluster)  [unwired: 1 in, 2 out]
              }
            }
          }
        }
        n74 = call <vilib>:"Add State(s) to Queue__jki_lib_state_machine.vi"("State(s) in (\"\")"=w165) -> ("States Out"=w164:string)  [unwired: 14 in]
      }
      frame "---------- Macro ----------" {
        # "Do not put any code in this frame.\n(It is a separator no-op. You can make a copy of this frame to create a new Macro frame)"
        n75 = call <vilib>:"Add State(s) to Queue__jki_lib_state_machine.vi"("State(s) in (\"\")"=w191) -> ("States Out"=w190:string)  [unwired: 14 in]
      }
      frame "Macro: Initialize" {
        # "Initialization Macro\n(This is called once, when the VI starts)"
        n76 = call <vilib>:"Add State(s) to Queue__jki_lib_state_machine.vi"("State(s) in Front (\"\")"="Data: Initialize\nInitialize Core Data\nUI: Initialize\nUI: Front Panel State >> Open", "State(s) in (\"\")"=w196) -> ("States Out"=w195:string)  [unwired: 13 in]
      }
      frame "Macro: Exit" {
        # "Exit Macro\n(This is called once, when the VI exits)"
        n77 = Unbundle By Name(w206) -> ("Core.Close Panel on Exit?"=w205:bool)
        n78 = Release Queue(queue=w198, force destroy? (F)=TRUE) -> (error out=w197:errorcluster)  [unwired: 1 in, 2 out]
        n79 = call <vilib>:"Clear Errors.vi"("error in (no error)"=w197) -> ()  [unwired: 5 in, 2 out]
        n80 = Select(t="UI: Front Panel State >> Close", s=w205, f="") -> (s? t:f=w202:string)
        n81 = call <vilib>:"Add State(s) to Queue__jki_lib_state_machine.vi"("State(s) in (\"\")"=w202, "State(s) at Back (\"\")"="Data: Cleanup\nExit") -> ("States Out"=w200:string)  [unwired: 13 in]
        n82 = call <vilib>:"Add State(s) to Queue__jki_lib_state_machine.vi"("State(s) in Front (\"\")"=w200, "State(s) in (\"\")"=w209) -> ("States Out"=w208:string)  [unwired: 13 in]
      }
      frame "---------- New Category ----------" {
        # "Template Separator\n(You can make a copy of, or modify, this frame)"
        n83 = call <vilib>:"Add State(s) to Queue__jki_lib_state_machine.vi"("State(s) in (\"\")"=w213) -> ("States Out"=w212:string)  [unwired: 14 in]
      }
      frame "Obsolete" {
        # "Your code here.\n(You can make a copy of, or modify, this frame)"
        n84 = Unbundle By Name(w222) -> ("Tik2"=w215:u32)
        n85 = Tick Count (ms)() -> (millisecond timer value=w217:u32)
        n86 = Subtract(x=w217, y=w215) -> (x-y=w220:u32)
        n87 = Greater?(x=w220, y=2000) -> (0:w218:bool)
        n88 = case shown="True" w218 {
          tunnel: w217 -> [_ w228]
          tunnel: [w226 w228] -> w216
          tunnel: w215 -> [w226 _]
          tunnel: [_ ""] -> w214
          frame False {
          }
          frame True {
          }
        }
        n89 = Bundle By Name(cluster=w222, "Tik2"=w216) -> (w221:T5)
        n90 = call <vilib>:"Add State(s) to Queue__jki_lib_state_machine.vi"("State(s) in Front (\"\")"=w214, "State(s) in (\"\")"=w225) -> ("States Out"=w224:string)  [unwired: 13 in]
      }
      frame "Action: Trig on" {
        (unwired) "fire>>force" ("Value (Signaling)")
        n91 = call <vilib>:"Add State(s) to Queue__jki_lib_state_machine.vi"("State(s) in (\"\")"=w232) -> ("States Out"=w231:string)  [unwired: 14 in]
      }
    }
  }
  n92 = call <userlib>:"Fit VI window to Largest Dec__ogtk.vi"() -> ()  [unwired: 6 in, 2 out]
